vi "JSONtext Tree VI.vi"   [LabVIEW 2017]
uses:
  JSONtext.lvlib
  7d68aa8f-9b87-40b7-8af7-862b2cb577a7.vi
  da5b140b-1f31-47a7-99bb-d9ea94cb1362.vi
  92dfa085-a272-46b9-9b4f-40831fb46b91.vi
  759eb72c-cd9a-46ab-b18b-586ecd80497b.vi
  b8ede321-213f-4692-b604-bb20c7ca9430.vi
  a061a676-e82d-4262-b343-6024fdc891cf.vi
  8e5c4d42-6327-4ad2-9cd5-39f5d411e4f9.vi
  074d6a8c-c26b-4d9f-b460-5b23c3205235.vi
  From JSON Text (string).vi
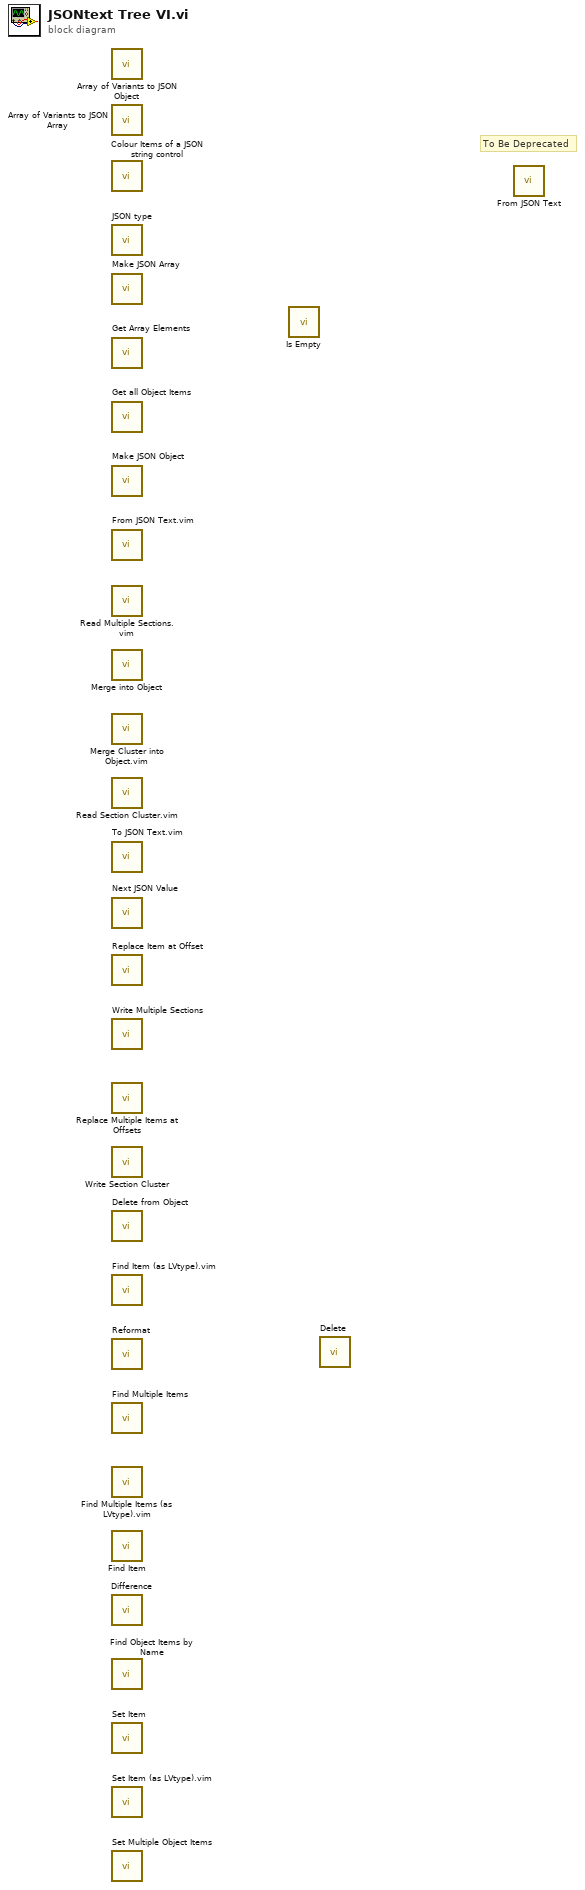
[diagram p0: block diagram]
diagram:
  # "To Be Deprecated"
  n1 = call "Array of Variants to JSON Object.vi"() -> ()  [unwired: 10 in, 2 out]
  n2 = call "Array of Variants to JSON Array.vi"() -> ()  [unwired: 10 in, 2 out]
  n3 = call "Colour Items of a JSON string control.vi"() -> ()  [unwired: 12 in]
  n4 = call "JSON type.vi"() -> ()  [unwired: 10 in, 2 out]
  n5 = call "Make JSON Array.vi"() -> ()  [unwired: 10 in, 2 out]
  n6 = call "Get Array Elements.vi"() -> ()  [unwired: 9 in, 3 out]
  n7 = call "Get all Object Items.vi"() -> ()  [unwired: 8 in, 4 out]
  n8 = call "Make JSON Object.vi"() -> ()  [unwired: 10 in, 2 out]
  n9 = call "From JSON Text.vim"() -> ()  [unwired: 10 in, 2 out]
  n10 = call "Read Multiple Sections.vim"() -> ()  [unwired: 9 in, 2 out]
  n11 = call "Merge into Object.vi"() -> ()  [unwired: 9 in, 2 out]
  n12 = call "Merge Cluster into Object.vim"() -> ()  [unwired: 9 in, 2 out]
  n13 = call "Read Section Cluster.vim"() -> ()  [unwired: 8 in, 3 out]
  n14 = call "To JSON Text.vim"() -> ()  [unwired: 10 in, 2 out]
  n15 = call "Next JSON Value.vi"() -> ()  [unwired: 8 in, 4 out]
  n16 = call "Replace Item at Offset.vi"() -> ()  [unwired: 10 in, 2 out]
  n17 = call "Write Multiple Sections.vi"() -> ()  [unwired: 9 in, 2 out]
  n18 = call "Replace Multiple Items at Offsets.vi"() -> ()  [unwired: 10 in, 2 out]
  n19 = call "Write Section Cluster.vi"() -> ()  [unwired: 9 in, 2 out]
  n20 = call "Delete from Object.vi"() -> ()  [unwired: 7 in, 4 out]
  n21 = call "Find Item (as LVtype).vim"() -> ()  [unwired: 8 in, 4 out]
  n22 = call "Reformat.vi"() -> ()  [unwired: 8 in, 4 out]
  n23 = call "Find Multiple Items.vi"() -> ()  [unwired: 8 in, 4 out]
  n24 = call "Find Multiple Items (as LVtype).vim"() -> ()  [unwired: 8 in, 4 out]
  n25 = call "Find Item.vi"() -> ()  [unwired: 8 in, 4 out]
  n26 = call "Difference.vi"() -> ()  [unwired: 9 in, 2 out]
  n27 = call "Find Object Items by Name.vi"() -> ()  [unwired: 9 in, 3 out]
  n28 = call "Set Item.vi"() -> ()  [unwired: 8 in, 3 out]
  n29 = call "Set Item (as LVtype).vim"() -> ()  [unwired: 8 in, 3 out]
  n30 = call "Set Multiple Object Items.vi"() -> ()  [unwired: 9 in, 2 out]
  n31 = call "Is Empty.vi"() -> ()  [unwired: 5 in, 1 out]
  n32 = call "Delete.vi"() -> ()  [unwired: 7 in, 4 out]
  n33 = call-poly "From JSON Text.vi"() -> ()  [unwired: 9 in, 3 out]
